vi "Fuel Injector Stage Transition.vi"(8 "error in (no error)":errorcluster, 11 "Node Ptr":T2 format="%.0x") -> (0 "error out":errorcluster)   [LabVIEW 2015, in "Fuel Injector Analysis Addon System Explorer.lvlib"]
uses:
  Fuel Injector Analysis Addon System Explorer.lvlib
  <vilib>/NI Veristand/Custom Device API/Custom Device Item Ref.ctl
  Shared/Types/Stage.Transition.Types.ctl
  <vilib>/NI Veristand/Custom Device API/Custom Device API.lvlib
  Shared/Fuel Injector Analysis Addon Shared.lvlib
panel:
  out "Units":string
  in  "Level":dbl
  in  "Stage Transition Setting":T1
  in  "SHDocVw.IWebBrowser":refnum<k7>(container)
  in  "Header":cluster{"Section Name":string}={"Section Name"="Custom Device Item Settings"}
  in  "Description":string
  out "Name":string
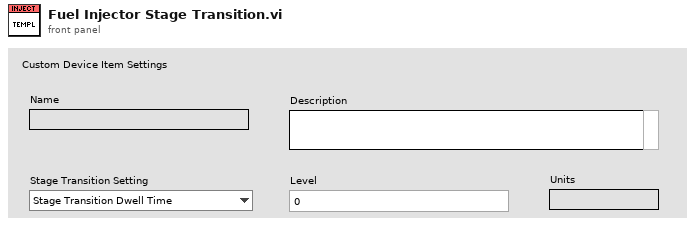
[diagram p1: front panel]
types:
  T1 = typedef "Fuel Injector Analysis Addon Shared.lvlib/Stage.Transition.Types.ctl" = enum8{"Stage Transition Dwell Time", "Stage Transition Voltage Level", "Stage Transition Current Drop", "Stage Transition Active Time"}
  T2 = typedef "Custom Device API.lvlib/Custom Device Item Ref.ctl" = u64
  T3 = typedef "Custom Device API.lvlib/Custom Device Channel.ctl" = cluster{"Type":T4, "Units":string, "Default Value":dbl, "Faultable":bool, "Scalable":bool}
  T4 = typedef "Custom Device API.lvlib/Custom Device Channel Type.ctl" = enum16{"Input", "Output"}
  T5 = typedef "Custom Device API.lvlib/Custom Device Commands.ctl" = enum16{"Default", "Item renamed", "Shutdown", "Dynamic button pressed"}
  T6 = typedef "Custom Device API.lvlib/Custom Device Item Info.ctl" = cluster{"Name":string, "Is Channel":bool, "GUID":string, "Is Waveform":bool}
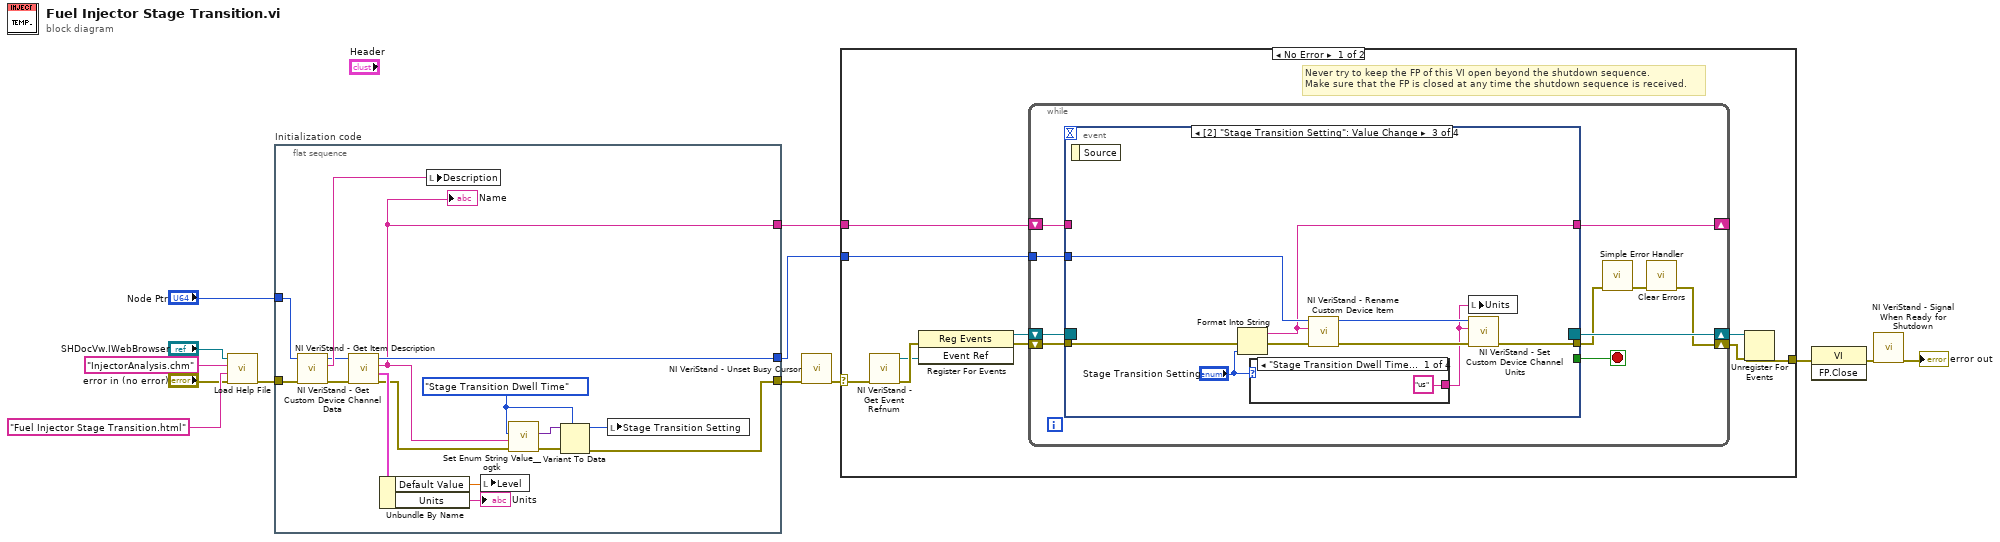
[diagram p0: block diagram]
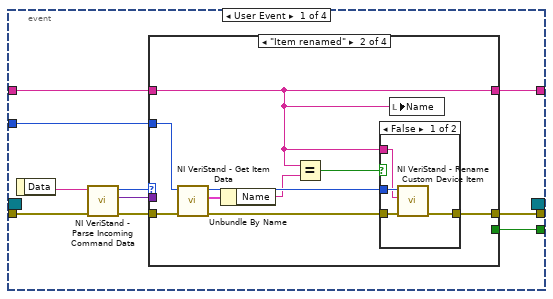
[diagram p2: hidden frame]
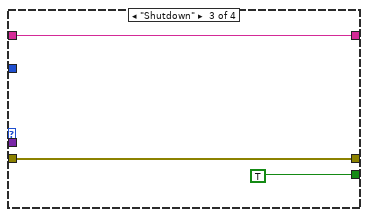
[diagram p5: hidden frame]
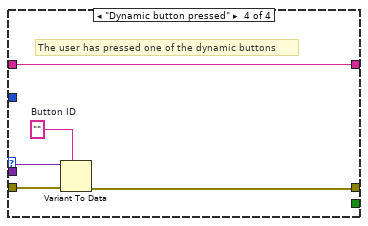
[diagram p6: hidden frame]
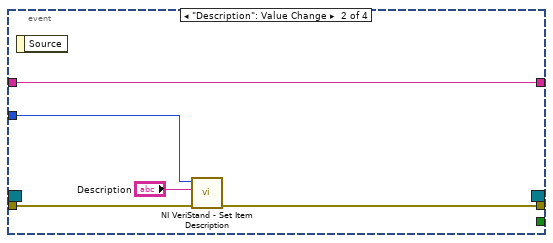
[diagram p7: hidden frame]
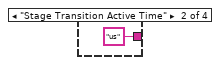
[diagram p8: hidden frame]
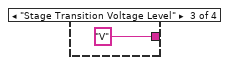
[diagram p9: hidden frame]
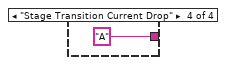
[diagram p10: hidden frame]
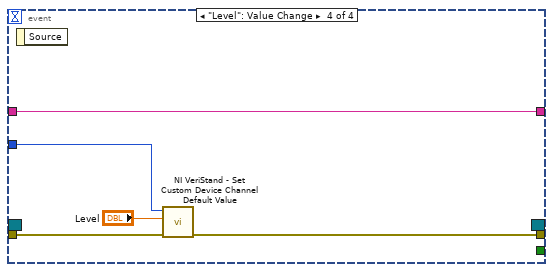
[diagram p11: hidden frame]
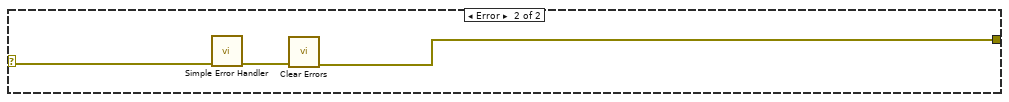
[diagram p12: hidden frame]
diagram:
  n1 = call "Load Help File.vi"("error in (no error)"="error in (no error)", "HTML File"="Fuel Injector Stage Transition.html", "Main CHM File"="InjectorAnalysis.chm", "SHDocVw.IWebBrowser2"="SHDocVw.IWebBrowser") -> ("error out"=w4:errorcluster)  [unwired: 7 in]
  n2 = flat-sequence "Initialization code" {
    tunnel: w4 -> [w29]
    tunnel: [w17] -> w10
    tunnel: [w26] -> w8
    tunnel: "Node Ptr" -> [w27]
    tunnel: [w16] -> w1
    frame #0 {
      w15 = Stage.Transition.Types."Stage Transition Dwell Time" ("Stage Transition Setting")
      n3 = call <vilib>:"NI VeriStand - Get Item Description.vi"("error in (no error)"=w29, "Item Ref in"=w27) -> ("error out"=w25:errorcluster, "Description"=w28:string, "Item Ref out"=w24:T2)  [unwired: 7 out]
      n4 = call <vilib>:"NI VeriStand - Get Custom Device Channel Data.vi"("error in (no error)"=w25, "Channel Ref in"=w24) -> ("error out"=w18:errorcluster, "Channel"=w23:T3, "Channel Name"=w16:string, "Channel Ref out"=w26:T2)  [unwired: 4 in, 2 out]
      "Name" <- w16
      n5 = Unbundle By Name(w23) -> ("Default Value"=w21:dbl, "Units"=→"Units":string)
      n6 = local write "Description"(w28) -> ()
      n7 = local write "Level"(w21) -> ()
      n8 = call <userlib>:"Set Enum String Value__ogtk.vi"("error in (no error)"=w18, "String Value"=w16, "Default Enum Value"=w15) -> ("error out"=w20:errorcluster, "Enum"=w19:variant)  [unwired: 7 in]
      n9 = Variant To Data(error in=w20, type=w15, Variant=w19) -> (data=w14:T1, error out=w17:errorcluster)
      n10 = local write "Stage Transition Setting"(w14) -> ()
    }
  }
  n11 = call <vilib>:"NI VeriStand - Unset Busy Cursor.vi"("error in (no error)"=w10) -> ("error out"=w9:errorcluster)  [unwired: 10 out]
  n12 = case shown="No Error" w9 {
    selector: w9 -> [w31 w109]
    tunnel: [w36 w107] -> w13
    tunnel: w8 -> [w32 _]
    tunnel: w1 -> [w30 _]
    frame No Error {
      # "Never try to keep the FP of this VI open beyond the shutdown sequence.\nMake sure that the FP is closed at any time the shutdown sequence is received."
      n13 = call <vilib>:"NI VeriStand - Get Event Refnum.vi"("error in (no error)"=w31) -> ("error out"=w39:errorcluster, "Event Ref"=w35:refnum<user-event>)  [unwired: 9 out]
      n14 = register-events(error in=w39, w35) -> (reference out=w33:refnum<event-registration>, error out=w34:errorcluster)  [unwired: 1 in]
      n15 = while {
        tunnel: w32 -> [w45]
        shift-right: [w42] -> w37
        shift-left: w34 -> [w48]
        shift-right: [w49] -> w38
        shift-left: w33 -> [w47]
        shift-right: [w40] -> _
        shift-left: w30 -> [w41]
        stop <- w46 stop-if-true
        n16 = event shown="[2] \"Stage Transition Setting\": Value Change" {
          selector: w47 -> [_ _ _ _]
          dyn-events: [_ _ _ _] -> w49
          timeout: _ -> [_ _ _ _]
          tunnel: w48 -> [w59 w87 w96 w106]
          tunnel: [w55 _ _ _] -> w46
          tunnel: [w54 w86 w91 w105] -> w44
          tunnel: w45 -> [w53 w88 w97 w103]
          tunnel: w41 -> [w51 w84 _ w102]
          tunnel: [w50 w84 w89 w102] -> w40
          event User Event {
            n17 = event-data() -> ("Data"=w58:string)  [unwired: 1 out]
            n18 = call <vilib>:"NI VeriStand - Parse Incoming Command Data.vi"("error in (no error)"=w59, "Incoming data"=w58) -> ("error out"=w57:errorcluster, "Outgoing data"=w52:variant, "Action"=w56:T5)  [unwired: 7 out]
            n19 = case shown="\"Item renamed\"" w56 {
              tunnel: w57 -> [w61 w67 w77 w83]
              tunnel: [_ _ TRUE _] -> w55
              tunnel: [w61 w70 w77 w80] -> w54
              tunnel: w53 -> [_ w68 _ _]
              tunnel: w52 -> [_ _ _ w82]
              tunnel: w51 -> [w60 w62 w76 w79]
              tunnel: [w60 w62 w76 w79] -> w50
              frame "Default", Default {
              }
              frame "Item renamed" {
                n20 = call <vilib>:"NI VeriStand - Get Item Data.vi"("error in (no error)"=w67, "Item Ref in"=w68) -> ("error out"=w66:errorcluster, "Item Info"=w69:T6, "Item Ref out"=w65:T2)  [unwired: 7 out]
                n21 = Unbundle By Name(w69) -> ("Name"=w64:string)
                n22 = Equal?(x=w62, y=w64) -> (x = y?=w63:bool)
                n23 = case shown="False" w63 {
                  tunnel: [w74 w75] -> w70
                  tunnel: w66 -> [w73 w75]
                  tunnel: w65 -> [w72 _]
                  tunnel: w62 -> [w71 _]
                  frame False {
                    n24 = call <vilib>:"NI VeriStand - Rename Custom Device Item.vi"("error in (no error)"=w73, "New Name"=w71, "Item Ref in"=w72) -> ("error out"=w74:errorcluster)  [unwired: 6 in, 2 out]
                  }
                  frame True {
                  }
                }
                n25 = local write "Name"(w62) -> ()
              }
              frame "Shutdown" {
              }
              frame "Dynamic button pressed" {
                w81 = ""  # Button ID
                # "The user has pressed one of the dynamic buttons"
                n26 = Variant To Data(error in=w83, type=w81, Variant=w82) -> (error out=w80:errorcluster)  [unwired: 1 out]
              }
            }
          }
          event "Description": Value Change {
            n27 = event-data() -> ()  [unwired: 2 out]
            n28 = call <vilib>:"NI VeriStand - Set Item Description.vi"("error in (no error)"=w87, "Description"="Description", "Item Ref in"=w88) -> ("error out"=w86:errorcluster)  [unwired: 8 out]
          }
          event Value Change {
            n29 = event-data() -> ()  [unwired: 2 out]
            n30 = Format Into String(error in=w96, "Stage Transition Setting") -> (resulting string=w89:string, error out=w95:errorcluster)  [unwired: 2 in]
            n31 = case shown="\"Stage Transition Dwell Time\"" "Stage Transition Setting" {
              tunnel: ["us" ("Units") "us" ("Units") "V" ("Units") "A" ("Units")] -> w90
              frame "Stage Transition Dwell Time" {
              }
              frame "Stage Transition Active Time" {
              }
              frame "Stage Transition Voltage Level" {
              }
              frame "Stage Transition Current Drop" {
              }
            }
            n32 = call <vilib>:"NI VeriStand - Rename Custom Device Item.vi"("error in (no error)"=w95, "New Name"=w89, "Item Ref in"=w97) -> ("error out"=w94:errorcluster, "Item Ref out"=w93:T2)  [unwired: 6 in, 1 out]
            n33 = local write "Units"(w90) -> ()
            n34 = call <vilib>:"NI VeriStand - Set Custom Device Channel Units.vi"("error in (no error)"=w94, "Units"=w90, "Channel Ref in"=w93) -> ("error out"=w91:errorcluster)  [unwired: 7 in, 1 out]
          }
          event "Level": Value Change {
            n35 = event-data() -> ()  [unwired: 2 out]
            n36 = call <vilib>:"NI VeriStand - Set Custom Device Channel Default Value.vi"("error in (no error)"=w106, "Default Value"="Level", "Channel Ref in"=w103) -> ("error out"=w105:errorcluster)  [unwired: 7 in, 1 out]
          }
        }
        n37 = call <vilib>:"Simple Error Handler.vi"("error in (no error)"=w44) -> ("error out"=w43:errorcluster)  [unwired: 1 in, 7 out]
        n38 = call <vilib>:"Clear Errors.vi"("error in (no error)"=w43) -> ("error out"=w42:errorcluster)  [unwired: 1 in, 5 out]
      }
      n39 = Unregister For Events(event registration refnum=w38, error in=w37) -> (error out=w36:errorcluster)
    }
    frame Error {
      n40 = call <vilib>:"Simple Error Handler.vi"("error in (no error)"=w109) -> ("error out"=w108:errorcluster)  [unwired: 1 in, 7 out]
      n41 = call <vilib>:"Clear Errors.vi"("error in (no error)"=w108) -> ("error out"=w107:errorcluster)  [unwired: 1 in, 5 out]
    }
  }
  n42 = invoke class="VI" method="FP.Close"(error in=w13) -> (error out=w12:errorcluster)  [unwired: 2 in, 2 out]
  n43 = call <vilib>:"NI VeriStand - Signal When Ready for Shutdown.vi"("error in (no error)"=w12) -> ("error out"=→"error out":errorcluster)  [unwired: 10 out]
